vi "Launcher.vi"   [LabVIEW 2017]
uses:
  UserEvents/StopUE.lvlib
  CodeModules/ErrorHandler/ErrorHandler.lvlib
  CodeModules/Controller/Controller.lvlib
  CodeModules/UserInterface/UserInterface.lvlib
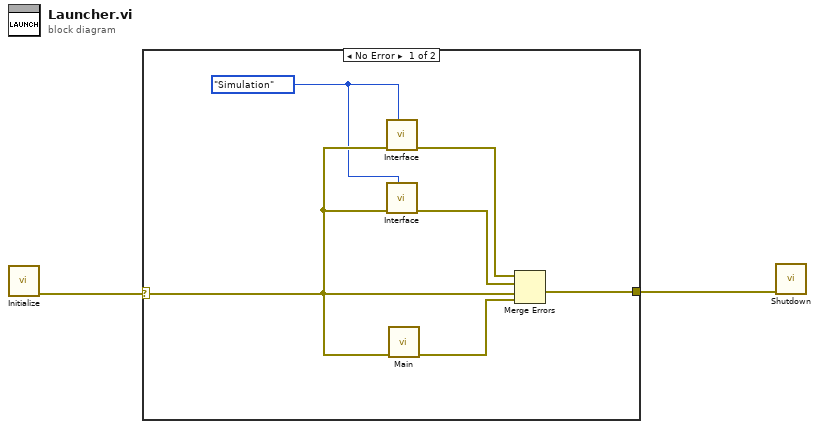
[diagram p0: block diagram]
diagram:
  n1 = call "Initialize.vi"() -> ("Error Out"=w1:errorcluster)  [unwired: 11 in]
  n2 = case shown="No Error" w1 {
    selector: w1 -> [w6 w9]
    tunnel: [w8 w9] -> w2
    frame No Error {
      w3 = enum16{"Simulation", "Embedded"}."Simulation" ("Interface")
      n3 = call "Interface.vi"("Interface"=w3, "Error In"=w6) -> ("Error Out"=w5:errorcluster)  [unwired: 9 in]
      n4 = call "Interface.vi"("Interface"=w3, "Error In"=w6) -> ("Error Out"=w4:errorcluster)  [unwired: 9 in]
      n5 = call "Main.vi"("Error In"=w6) -> ("Error Out"=w7:errorcluster)  [unwired: 10 in]
      n6 = Merge Errors(w5, w4, w6, w7) -> (w8:errorcluster)
    }
    frame Error {
    }
  }
  n7 = call "Shutdown.vi"("Error In"=w2) -> ()  [unwired: 10 in, 1 out]
